vi "Set Ref Clk.vi"(6 "Action":enum16{"Initialize", "Set Ref Clk"}(ring), 8 "error in (no error)":errorcluster, 11 "task in":refnum<k21>) -> (0 "error out":errorcluster, 3 "task out":refnum<k21>)   [LabVIEW 2015]
uses:
  <resource>/objmgr/daqmx.rc
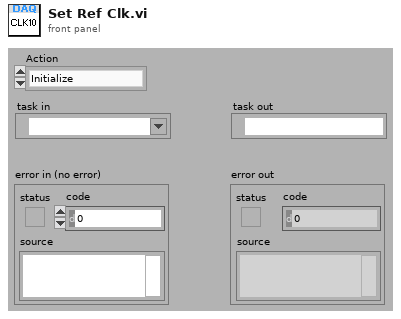
[diagram p1: front panel]
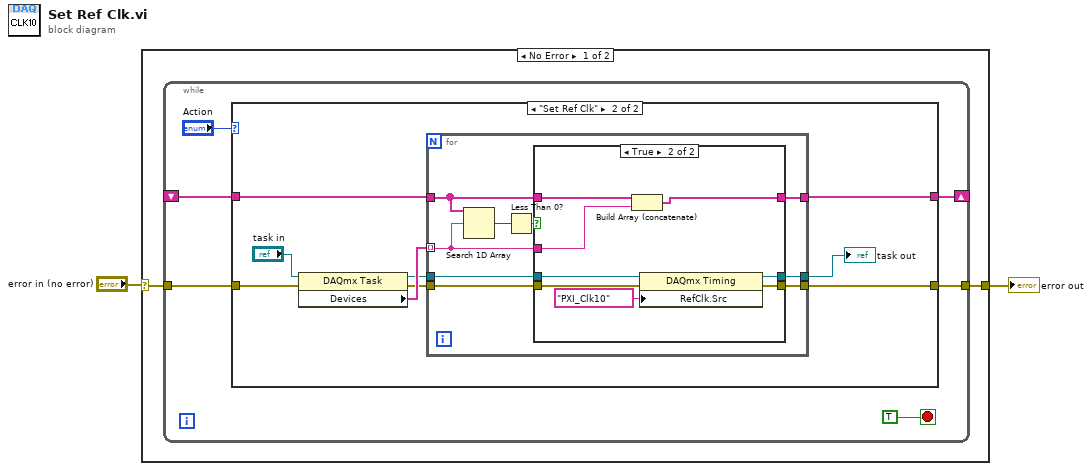
[diagram p0: block diagram]
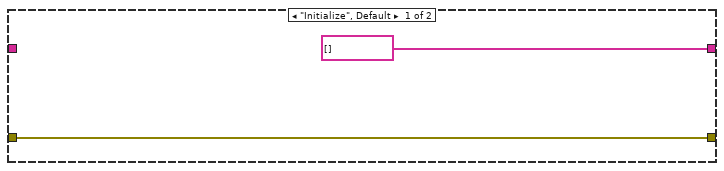
[diagram p2: hidden frame]
diagram:
  n1 = case shown="No Error" "error in (no error)" {
    selector: "error in (no error)" -> [w4 w42]
    tunnel: [w3 w42] -> w1
    frame No Error {
      n2 = while {
        tunnel: w4 -> [w9]
        tunnel: [w8] -> w3
        shift-right: [w6] -> _
        shift-left: _ -> [w5]
        stop <- TRUE stop-if-true
        n3 = case shown="\"Set Ref Clk\"" "Action" {
          tunnel: [w12 w14] -> w8
          tunnel: w9 -> [w12 w20]
          tunnel: [tag[] [] ("DevNames") w15] -> w6
          tunnel: w5 -> [_ w16]
          frame "Initialize", Default {
          }
          frame "Set Ref Clk" {
            n4 = property class="DAQmx Task"(reference="task in", error in=w20) -> (reference out=w18:refnum<k21>, error out=w17:errorcluster, "Devices"=w19:tag[])
            n5 = for {
              tunnel: w19 -> [w23] mode=indexing
              tunnel: w18 -> [w28]
              tunnel: w17 -> [w27]
              tunnel: w16 -> [w26]
              tunnel: [w25] -> w15
              tunnel: [w24] -> w14
              tunnel: [w22] -> w13
              n6 = Search 1D Array(1D array=w26, element=w23) -> (index of element=w30:i32)  [unwired: 1 in]
              n7 = Less Than 0?(x=w30) -> (x < 0?=w29:bool)
              n8 = case shown="True" w29 {
                tunnel: w28 -> [w31 w40]
                tunnel: w27 -> [w32 w41]
                tunnel: [w32 w38] -> w24
                tunnel: w26 -> [w33 w37]
                tunnel: [w33 w35] -> w25
                tunnel: w23 -> [_ w36]
                tunnel: [w31 w34] -> w22
                frame False {
                }
                frame True {
                  n9 = Build Array (concatenate)(w37, w36) -> (w35:tag[])
                  n10 = property class="DAQmx Timing"(reference=w40, error in=w41, "RefClk.Src"=tag "PXI_Clk10") -> (reference out=w34:refnum<k21>, error out=w38:errorcluster)
                }
              }
            }
            "task out" <- w13
          }
        }
      }
    }
    frame Error {
    }
  }
  "error out" <- w1
